vi "Begin.vi"(8 "error in":errorcluster) -> (0 "error out":errorcluster)   [LabVIEW 2020]
doc: "Called before other user functions, this VI is expected to open initial I/O refnums, load in file data, and do all program initialization. Notice that the <B>error out</B> terminal is simply used for data flow. Wiring it to other structures or subVIs ensures that this VI runs first."
uses:
  <vilib>/Rock Robotics/SystemInterfaces/DIO/FPGA_DIOPWMChannel.ctl
  <vilib>/Rock Robotics/WPI/SafetyOutput/WPI_SafetyOutputConfigMenu.ctl
  <vilib>/Rock Robotics/WPI/DriverStation/WPI_DriverStationRobotMode2.ctl
  <vilib>/Rock Robotics/WPI/Joystick/WPI_JoystickDeviceEnum.ctl
  Robot Global Data.vi
  <vilib>/Rock Robotics/Network Tables/NT Write String Array.vi
  <vilib>/Rock Robotics/WPI/RobotDrive/WPI_RobotDriveOpen2MotorWithVictorSPX.vi
  <vilib>/Rock Robotics/WPI/ThirdParty/Phoenix-LabVIEW/Motor Controller/Controls/CTRE_Phoenix_MotorControl_NeutralMode.ctl
  <vilib>/Rock Robotics/SystemInterfaces/DIO/FPGA_DIOChannel.ctl
  <vilib>/Rock Robotics/WPI/PWM/WPI_PWMDeadband.ctl
  <vilib>/Rock Robotics/WPI/MotorControl/WPI_MotorControlType.ctl
  <vilib>/Rock Robotics/WPI/MotorControl/WPI_MotorControlDeviceRef.ctl
  <vilib>/Rock Robotics/WPI/RobotDrive/WPI_RobotDriveDevRef.ctl
  <vilib>/Rock Robotics/WPI/ThirdParty/Phoenix-LabVIEW/Motor Controller/Controls/CTRE_Phoenix_MotorControl_FeedbackDevice.ctl
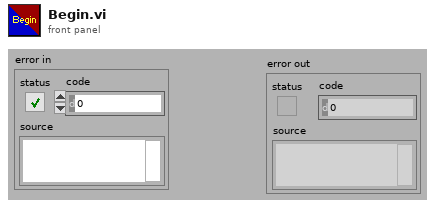
[diagram p1: front panel]
types:
  T1 = typedef "CTRE_Phoenix_MotorControl_FeedbackDevice.ctl" = i8
  T2 = typedef "CTRE_Phoenix_MotorControl_NeutralMode.ctl" = enum8{"EEPROMSetting", "Override to Coast", "Override to Brake"}
  T3 = typedef "WPI_SafetyOutputConfigMenu.ctl" = enum16{"Enable", "Disable"}
  T4 = typedef "WPI_RobotDriveDevRef.ctl" = cluster{"DevStatus":errorcluster, "Motors[]":T5[], "Square Inputs":bool, "Max Output":dbl}
  T5 = typedef "WPI_MotorControlDeviceRef.ctl" = cluster{"DeviceStatus":errorcluster, "Type":T6, "PWM":cluster{"PWM Channel":T7, "DeadBand":T8}, "CAN":cluster{"Device Number":u8, "SetOutput VI Ref":variant, "GetOutput VI Ref":variant, "Enable VI Ref":variant, "Disable VI Ref":variant, "Data":variant}, "Invert":bool, "DIO PWM":cluster{"PWM \"Enable\" Channel":T7, "DIOChannel":T9, "PWM Rate":dbl}}
  T6 = typedef "WPI_MotorControlType.ctl" = enum16{"PWM", "CAN", "DIO PWM"}
  T7 = typedef "FPGA_DIOPWMChannel.ctl" = enum8{"PWM 0", "PWM 1", "PWM 2", "PWM 3", "PWM 4", "PWM 5", "PWM 6", "PWM 7", "PWM 8", "PWM 9", "PWM MXP 0", "PWM MXP 1", "PWM MXP 2", "PWM MXP 3", "PWM MXP 4", "PWM MXP 5", "PWM MXP 6", "PWM MXP 7", "PWM MXP 8", "PWM MXP 9", "Invalid"}
  T8 = typedef "WPI_PWMDeadband.ctl" = cluster{"Name":string, "maxPositivePwm":i32, "minPositivePwm":i32, "centerPwm":i32, "maxNegativePwm":i32, "minNegativePwm":i32, "angularRange":u16}
  T9 = typedef "FPGA_DIOChannel.ctl" = enum8{"DIO 0", "DIO 1", "DIO 2", "DIO 3", "DIO 4", "DIO 5", "DIO 6", "DIO 7", "DIO 8", "DIO 9", "DIO MXP 0", "DIO MXP 1", "DIO MXP 2", "DIO MXP 3", "DIO MXP 4", "DIO MXP 5", "DIO MXP 6", "DIO MXP 7", "DIO MXP 8", "DIO MXP 9", "DIO MXP 10", "DIO MXP 11", "DIO MXP 12", "DIO MXP 13", "DIO MXP 14", "DIO MXP 15", "SPI Port CS1", "SPI Port CS2", "SPI Port CS3", "SPI Port MISO", "SPI Port MOSI", "Invalid"}
  T10 = typedef "WPI_JoystickDeviceEnum.ctl" = enum16{"USB 0", "USB 1", "USB 2", "USB 3", "USB 4", "USB 5"}
  T11 = typedef "WPI_DriverStationRobotMode2.ctl" = enum16{"Autonomous Disabled", "Autonomous Enabled", "Teleop Disabled", "Teleop Enabled", "Disconnected", "Finish", "Test Disabled", "Test Enabled", "Emergency Stopped"}
  T12 = typedef "WPI_JoystickDevRef.ctl" = cluster{"Device":T10}
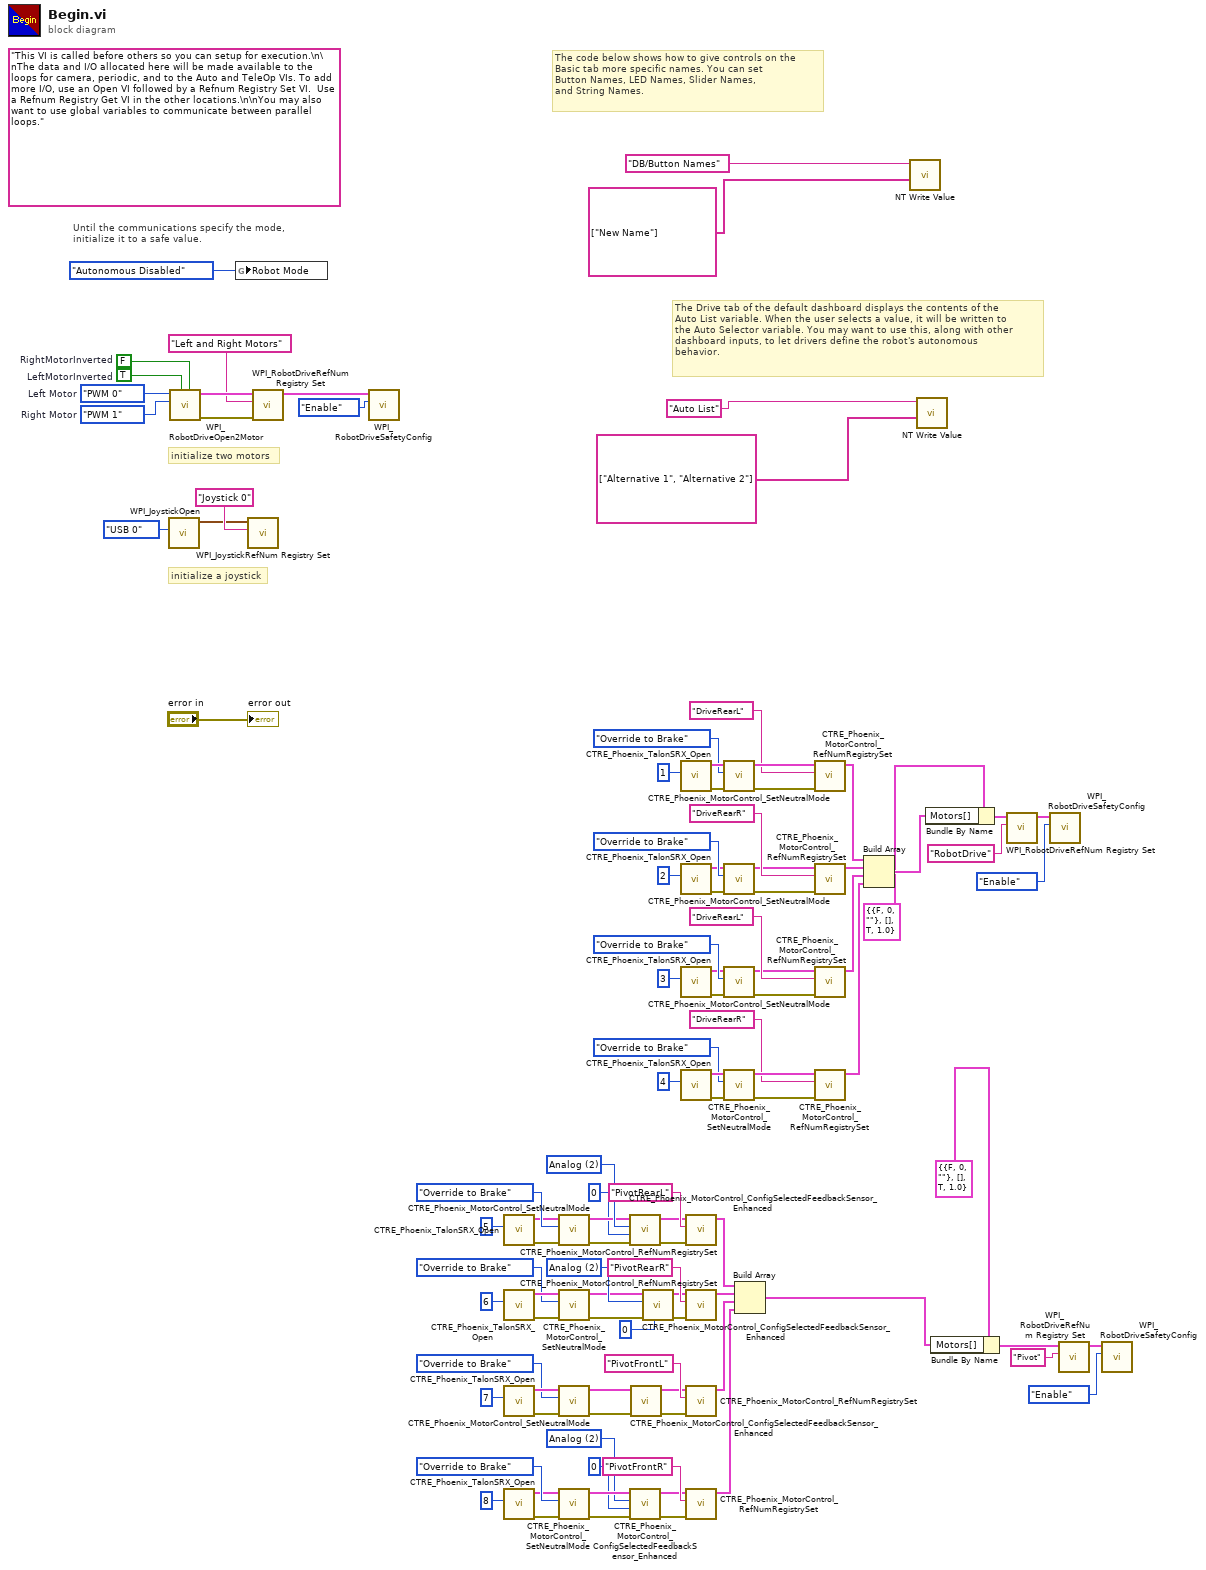
[diagram p0: block diagram]
diagram:
  w2 = T1 2 items=["QuadEncoder"=0, "Analog"=2, "Tachometer"=4, "Pulse Width Encoded Position"=8, "Sensor Sum (S0 + S1)"=9, "Sensor Difference (D0 - D1)"=10, "Remote Source 0"=11, "Remote Source 1"=12, "Software Emulated"=15] ("Feedback Device")
  w16 = T1 2 items=["QuadEncoder"=0, "Analog"=2, "Tachometer"=4, "Pulse Width Encoded Position"=8, "Sensor Sum (S0 + S1)"=9, "Sensor Difference (D0 - D1)"=10, "Remote Source 0"=11, "Remote Source 1"=12, "Software Emulated"=15] ("Feedback Device")
  w23 = T1 2 items=["QuadEncoder"=0, "Analog"=2, "Tachometer"=4, "Pulse Width Encoded Position"=8, "Sensor Sum (S0 + S1)"=9, "Sensor Difference (D0 - D1)"=10, "Remote Source 0"=11, "Remote Source 1"=12, "Software Emulated"=15] ("Feedback Device")
  (unwired) "This VI is called before others so you can setup for execution.\n\nThe data and I/O allocated here will be made available to the loops for camera, periodic, and to the Auto and TeleOp VIs. To add more I/O, use an Open VI followed by a Refnum Registry Set VI.  Use a Refnum Registry Get VI in the other locations.\n\nYou may also want to use global variables to communicate between parallel loops."
  w102 = FPGA_DIOPWMChannel."PWM 1"  # Right Motor
  w103 = FPGA_DIOPWMChannel."PWM 0"  # Left Motor
  w107 = TRUE  # LeftMotorInverted
  w108 = FALSE  # RightMotorInverted
  # "The Drive tab of the default dashboard displays the contents of the\nAuto List variable. When the user selects a value, it will be written to\nthe Auto Selector variable. You may want to use this, along with other\ndashboard inputs, to let drivers define the robot's autonomous\nbehavior."
  # "The code below shows how to give controls on the\nBasic tab more specific names. You can set\nButton Names, LED Names, Slider Names,\nand String Names."
  # "initialize a joystick"
  # "Until the communications specify the mode,\ninitialize it to a safe value."
  # "initialize two motors"
  n1 = call <vilib>:"WPI_JoystickOpen.vi"("JoystickDevice"=WPI_JoystickDeviceEnum."USB 0") -> ("JoystickDevRef"=w97:T12)  [unwired: 10 in]
  n2 = call-poly <vilib>:"WPI_RobotDriveOpen2Motor.vi"("Right Motor Inverted"=w108, "Left Motor Inverted"=w107, "Right Motor"=w102, "Left Motor"=w103) -> ("error out"=w104:errorcluster, "RobotDriveDevRef"=w106:T4)  [unwired: 1 in, 5 out]
  n3 = global write "Robot Global Data.vi" "Robot Mode"(WPI_DriverStationRobotMode2."Autonomous Disabled" ("Robot Mode")) -> ()
  n4 = call <vilib>:"WPI_JoystickRefNum Registry Set.vi"("refnum name"="Joystick 0", "JoystickDevRef"=w97) -> ()  [unwired: 8 in, 2 out]
  n5 = call <vilib>:"WPI_RobotDriveRefNum Registry Set.vi"("error in (no error)"=w104, "refnum name"="Left and Right Motors", "RobotDriveDevRef"=w106) -> ("RobotDriveDevRef"=w101:T4)  [unwired: 1 in, 7 out]
  n6 = call <vilib>:"WPI_RobotDriveSafetyConfig.vi"("mode"=WPI_SafetyOutputConfigMenu."Enable", "RobotDriveDevRef"=w101) -> ()  [unwired: 8 in, 2 out]
  n7 = call <vilib>:"CTRE_Phoenix_TalonSRX_Open.vi"("Device Number"=5) -> ("error out"=w19:errorcluster, "PhoenixMotorControlDevRef"=w69:T5)  [unwired: 9 in]
  n8 = call <vilib>:"CTRE_Phoenix_TalonSRX_Open.vi"("Device Number"=6) -> ("error out"=w43:errorcluster, "PhoenixMotorControlDevRef"=w42:T5)  [unwired: 9 in]
  n9 = call <vilib>:"CTRE_Phoenix_TalonSRX_Open.vi"("Device Number"=7) -> ("error out"=w33:errorcluster, "PhoenixMotorControlDevRef"=w32:T5)  [unwired: 9 in]
  n10 = call <vilib>:"CTRE_Phoenix_TalonSRX_Open.vi"("Device Number"=8) -> ("error out"=w36:errorcluster, "PhoenixMotorControlDevRef"=w37:T5)  [unwired: 9 in]
  n11 = call <vilib>:"CTRE_Phoenix_MotorControl_SetNeutralMode.vi"("error in (no error)"=w19, "Motor Control Neutral Mode"=CTRE_Phoenix_MotorControl_NeutralMode."Override to Brake", "PhoenixMotorControlDevRef"=w69) -> ("error out"=w18:errorcluster, "PhoenixMotorControlDevRef"=w22:T5)  [unwired: 7 in]
  n12 = call <vilib>:"CTRE_Phoenix_MotorControl_SetNeutralMode.vi"("error in (no error)"=w43, "Motor Control Neutral Mode"=CTRE_Phoenix_MotorControl_NeutralMode."Override to Brake", "PhoenixMotorControlDevRef"=w42) -> ("error out"=w13:errorcluster, "PhoenixMotorControlDevRef"=w14:T5)  [unwired: 7 in]
  n13 = call <vilib>:"CTRE_Phoenix_MotorControl_SetNeutralMode.vi"("error in (no error)"=w33, "Motor Control Neutral Mode"=CTRE_Phoenix_MotorControl_NeutralMode."Override to Brake", "PhoenixMotorControlDevRef"=w32) -> ("error out"=w8:errorcluster, "PhoenixMotorControlDevRef"=w10:T5)  [unwired: 7 in]
  n14 = call <vilib>:"CTRE_Phoenix_MotorControl_SetNeutralMode.vi"("error in (no error)"=w36, "Motor Control Neutral Mode"=CTRE_Phoenix_MotorControl_NeutralMode."Override to Brake", "PhoenixMotorControlDevRef"=w37) -> ("error out"=w5:errorcluster, "PhoenixMotorControlDevRef"=w6:T5)  [unwired: 7 in]
  n15 = call <vilib>:"CTRE_Phoenix_MotorControl_ConfigSelectedFeedbackSensor_Enhanced.vi"("error in (no error)"=w18, "pidLoopIdx"=0, "Feedback Device"=w23, "PhoenixMotorControlDevRef"=w22) -> ("error out"=w17:errorcluster, "PhoenixMotorControlDevRef"=w21:T5)  [unwired: 6 in]
  n16 = call <vilib>:"CTRE_Phoenix_MotorControl_ConfigSelectedFeedbackSensor_Enhanced.vi"("error in (no error)"=w5, "pidLoopIdx"=0, "Feedback Device"=w2, "PhoenixMotorControlDevRef"=w6) -> ("error out"=w3:errorcluster, "PhoenixMotorControlDevRef"=w4:T5)  [unwired: 6 in]
  n17 = call <vilib>:"CTRE_Phoenix_MotorControl_ConfigSelectedFeedbackSensor_Enhanced.vi"("error in (no error)"=w8, "PhoenixMotorControlDevRef"=w10) -> ("error out"=w7:errorcluster, "PhoenixMotorControlDevRef"=w9:T5)  [unwired: 8 in]
  n18 = call <vilib>:"CTRE_Phoenix_MotorControl_ConfigSelectedFeedbackSensor_Enhanced.vi"("timeoutMs"=u32 0, "error in (no error)"=w13, "Feedback Device"=w16, "PhoenixMotorControlDevRef"=w14) -> ("error out"=w11:errorcluster, "PhoenixMotorControlDevRef"=w12:T5)  [unwired: 6 in]
  n19 = call <vilib>:"CTRE_Phoenix_TalonSRX_Open.vi"("Device Number"=1) -> ("error out"=w87:errorcluster, "PhoenixMotorControlDevRef"=w86:T5)  [unwired: 9 in]
  n20 = call <vilib>:"CTRE_Phoenix_TalonSRX_Open.vi"("Device Number"=2) -> ("error out"=w62:errorcluster, "PhoenixMotorControlDevRef"=w63:T5)  [unwired: 9 in]
  n21 = call <vilib>:"CTRE_Phoenix_TalonSRX_Open.vi"("Device Number"=3) -> ("error out"=w48:errorcluster, "PhoenixMotorControlDevRef"=w49:T5)  [unwired: 9 in]
  n22 = call <vilib>:"CTRE_Phoenix_TalonSRX_Open.vi"("Device Number"=4) -> ("error out"=w55:errorcluster, "PhoenixMotorControlDevRef"=w54:T5)  [unwired: 9 in]
  n23 = call <vilib>:"CTRE_Phoenix_MotorControl_RefNumRegistrySet.vi"("error in (no error)"=w17, "refnum name"="PivotRearL", "PhoenixMotorControlDevRef"=w21) -> ("PhoenixMotorControlDevRef"=w75:T5)  [unwired: 7 in, 1 out]
  n24 = call <vilib>:"CTRE_Phoenix_MotorControl_RefNumRegistrySet.vi"("error in (no error)"=w11, "refnum name"="PivotRearR", "PhoenixMotorControlDevRef"=w12) -> ("PhoenixMotorControlDevRef"=w26:T5)  [unwired: 7 in, 1 out]
  n25 = call <vilib>:"CTRE_Phoenix_MotorControl_RefNumRegistrySet.vi"("error in (no error)"=w7, "refnum name"="PivotFrontL", "PhoenixMotorControlDevRef"=w9) -> ("PhoenixMotorControlDevRef"=w25:T5)  [unwired: 7 in, 1 out]
  n26 = call <vilib>:"CTRE_Phoenix_MotorControl_RefNumRegistrySet.vi"("error in (no error)"=w3, "refnum name"="PivotFrontR", "PhoenixMotorControlDevRef"=w4) -> ("PhoenixMotorControlDevRef"=w24:T5)  [unwired: 7 in, 1 out]
  n27 = call <vilib>:"CTRE_Phoenix_MotorControl_SetNeutralMode.vi"("error in (no error)"=w87, "Motor Control Neutral Mode"=CTRE_Phoenix_MotorControl_NeutralMode."Override to Brake", "PhoenixMotorControlDevRef"=w86) -> ("error out"=w89:errorcluster, "PhoenixMotorControlDevRef"=w88:T5)  [unwired: 7 in]
  n28 = call <vilib>:"CTRE_Phoenix_MotorControl_SetNeutralMode.vi"("error in (no error)"=w62, "Motor Control Neutral Mode"=CTRE_Phoenix_MotorControl_NeutralMode."Override to Brake", "PhoenixMotorControlDevRef"=w63) -> ("error out"=w60:errorcluster, "PhoenixMotorControlDevRef"=w61:T5)  [unwired: 7 in]
  n29 = call <vilib>:"CTRE_Phoenix_MotorControl_SetNeutralMode.vi"("error in (no error)"=w48, "Motor Control Neutral Mode"=CTRE_Phoenix_MotorControl_NeutralMode."Override to Brake", "PhoenixMotorControlDevRef"=w49) -> ("error out"=w46:errorcluster, "PhoenixMotorControlDevRef"=w47:T5)  [unwired: 7 in]
  n30 = call <vilib>:"CTRE_Phoenix_MotorControl_SetNeutralMode.vi"("error in (no error)"=w55, "Motor Control Neutral Mode"=CTRE_Phoenix_MotorControl_NeutralMode."Override to Brake", "PhoenixMotorControlDevRef"=w54) -> ("error out"=w57:errorcluster, "PhoenixMotorControlDevRef"=w56:T5)  [unwired: 7 in]
  n31 = Build Array(w75, w26, w25, w24) -> (w76:T5[])
  n32 = call <vilib>:"CTRE_Phoenix_MotorControl_RefNumRegistrySet.vi"("error in (no error)"=w89, "refnum name"="DriveRearL", "PhoenixMotorControlDevRef"=w88) -> ("PhoenixMotorControlDevRef"=w82:T5)  [unwired: 7 in, 1 out]
  n33 = call <vilib>:"CTRE_Phoenix_MotorControl_RefNumRegistrySet.vi"("error in (no error)"=w60, "refnum name"="DriveRearR", "PhoenixMotorControlDevRef"=w61) -> ("PhoenixMotorControlDevRef"=w29:T5)  [unwired: 7 in, 1 out]
  n34 = call <vilib>:"CTRE_Phoenix_MotorControl_RefNumRegistrySet.vi"("error in (no error)"=w46, "refnum name"="DriveRearL", "PhoenixMotorControlDevRef"=w47) -> ("PhoenixMotorControlDevRef"=w28:T5)  [unwired: 7 in, 1 out]
  n35 = call <vilib>:"CTRE_Phoenix_MotorControl_RefNumRegistrySet.vi"("error in (no error)"=w57, "refnum name"="DriveRearR", "PhoenixMotorControlDevRef"=w56) -> ("PhoenixMotorControlDevRef"=w27:T5)  [unwired: 7 in, 1 out]
  n36 = Build Array(w82, w29, w28, w27) -> (w81:T5[])
  n37 = call-poly <vilib>:"NT Write Value.vi"("String Array"=string[] ["New Name"], "Name"="DB/Button Names") -> ()  [unwired: 9 in, 1 out]
  n38 = call-poly <vilib>:"NT Write Value.vi"("String Array"=string[] ["Alternative 1", "Alternative 2"], "Name"="Auto List") -> ()  [unwired: 9 in, 1 out]
  n39 = Bundle By Name(cluster=T4 {"DevStatus"={"status"=FALSE, "code"=0, "source"=""}, "Motors[]"=[], "Square Inputs"=TRUE, "Max Output"=1.0} ("RobotDriveDevRef"), "Motors[]"=w81) -> (w66:T4)
  n40 = Bundle By Name(cluster=T4 {"DevStatus"={"status"=FALSE, "code"=0, "source"=""}, "Motors[]"=[], "Square Inputs"=TRUE, "Max Output"=1.0} ("RobotDriveDevRef"), "Motors[]"=w76) -> (w73:T4)
  n41 = call <vilib>:"WPI_RobotDriveRefNum Registry Set.vi"("refnum name"="RobotDrive", "RobotDriveDevRef"=w66) -> ("RobotDriveDevRef"=w80:T4)  [unwired: 8 in, 1 out]
  n42 = call <vilib>:"WPI_RobotDriveSafetyConfig.vi"("mode"=WPI_SafetyOutputConfigMenu."Enable", "RobotDriveDevRef"=w80) -> ()  [unwired: 8 in, 2 out]
  n43 = call <vilib>:"WPI_RobotDriveRefNum Registry Set.vi"("refnum name"="Pivot", "RobotDriveDevRef"=w73) -> ("RobotDriveDevRef"=w77:T4)  [unwired: 8 in, 1 out]
  n44 = call <vilib>:"WPI_RobotDriveSafetyConfig.vi"("mode"=WPI_SafetyOutputConfigMenu."Enable", "RobotDriveDevRef"=w77) -> ()  [unwired: 8 in, 2 out]
  "error out" <- "error in"
